vi "sub_vi_set_linear_parameters.vi"(5 "intercept":dbl, 7 "slope":dbl, 8 "error in (no error)":errorcluster, 10 "gain":i32, 11 "VISA resource name in":refnum<visa-resource-name>) -> (0 "error out":errorcluster, 3 "VISA resource name out":refnum<visa-resource-name>)   [LabVIEW 2019]
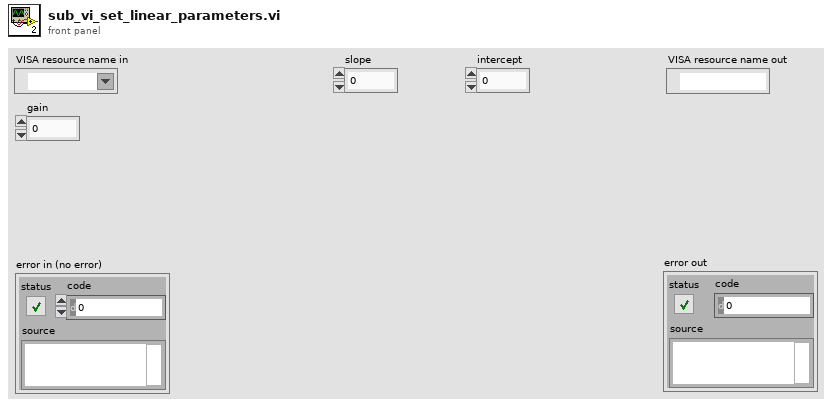
[diagram p1: front panel]
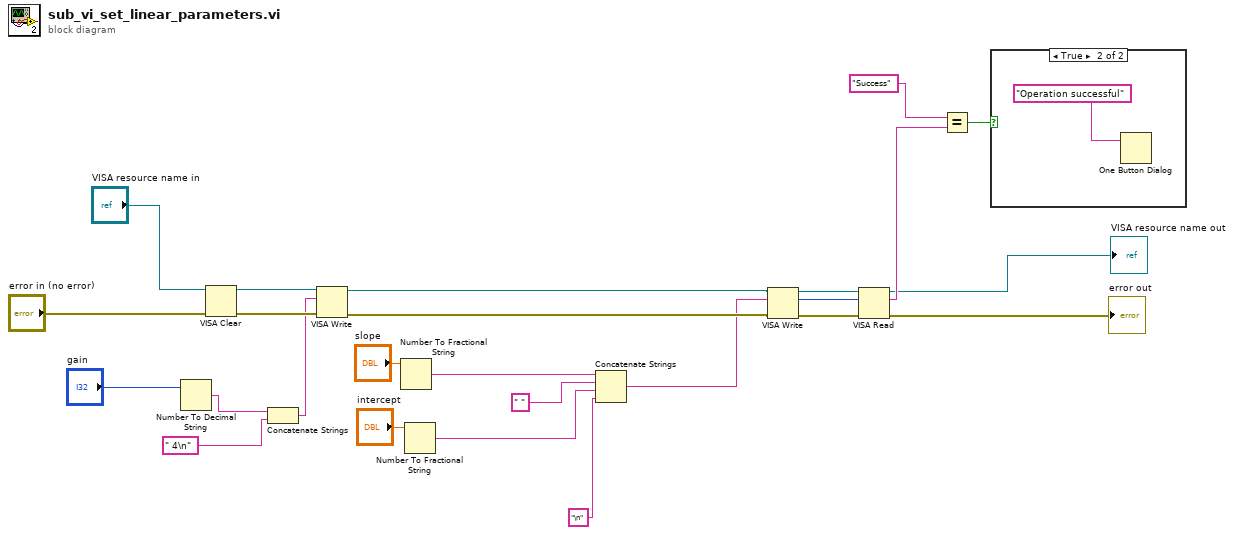
[diagram p0: block diagram]
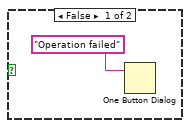
[diagram p2: hidden frame]
diagram:
  n1 = Number To Decimal String(number="gain") -> (decimal integer string=w18:string)  [unwired: 1 in]
  n2 = VISA Clear(VISA resource name="VISA resource name in", error in (no error)="error in (no error)") -> (VISA resource name out=w25:refnum<visa-resource-name>, error out=w24:errorcluster)
  n3 = Concatenate Strings(w18, " 4\n" ("string")) -> (w16:string)
  n4 = VISA Write(VISA resource name=w25, write buffer=w16, error in (no error)=w24) -> (VISA resource name out=w23:refnum<visa-resource-name>, error out=w22:errorcluster)  [unwired: 1 out]
  n5 = Number To Fractional String(number="slope") -> (F-format string=w13:string)  [unwired: 3 in]
  n6 = Number To Fractional String(number="intercept") -> (F-format string=w11:string)  [unwired: 3 in]
  n7 = Concatenate Strings(w13, " " ("string"), w11, "\n" ("string")) -> (w9:string)
  n8 = VISA Write(VISA resource name=w23, write buffer=w9, error in (no error)=w22) -> (VISA resource name out=w21:refnum<visa-resource-name>, return count=w1:u32, error out=w20:errorcluster)
  n9 = VISA Read(VISA resource name=w21, byte count=w1, error in (no error)=w20) -> (VISA resource name out=→"VISA resource name out":refnum<visa-resource-name>, read buffer=w6:string, error out=→"error out":errorcluster)  [unwired: 1 out]
  n10 = Equal?(x="Success" ("y"), y=w6) -> (x = y?=w8:bool)
  n11 = case shown="True" w8 {
    frame False {
      n12 = One Button Dialog(message="Operation failed") -> ()  [unwired: 1 in, 1 out]
    }
    frame True {
      n13 = One Button Dialog(message="Operation successful") -> ()  [unwired: 1 in, 1 out]
    }
  }
